vi "Sort Power Meters.vi"(0 "SG Path PM Accessor Base Array in":refnum<class "SG Path PM Accessor Base.lvclass">[](array[class]), 5 "Power Meter Base Array in":refnum<class "Power Meter Base.lvclass">[](array[class]), 11 "error in":errorcluster) -> (2 "All Present SG Path PMs Except Requested":refnum<class "SG Path PM Accessor Base.lvclass">[](array[class]), 3 "All Present PMs Except Requested":refnum<class "Power Meter Base.lvclass">[](array[class]), 4 "Requested SG Path PM Accessor":refnum<class "SG Path PM Accessor Base.lvclass">, 6 "Requested PM":refnum<class "Power Meter Base.lvclass">, 8 "Requested PM Found?":bool, 15 "error out":errorcluster)   [LabVIEW 2023, in "RFFixtureCharact.Instruments.lvlib" / "Power Meter Factory.lvclass"]
uses:
  Power Meter Factory.lvclass
  Power Meter Base/Power Meter Base.lvclass
  SG Path PM Accessor Base/SG Path PM Accessor Base.lvclass
  Power Meter Base/Power Meter Base.lvclass/Power Meter Base.ctl
  Power Meter Base/Properties/Write Active Instrument Info.vi
  Power Meter Base/Properties/Read Instrument Info Array.vi
  Common/Data Cache/Settings Dictionary/Setting Keys.vi
  Common/RFCalAndFixtureCharact.Common.lvlib
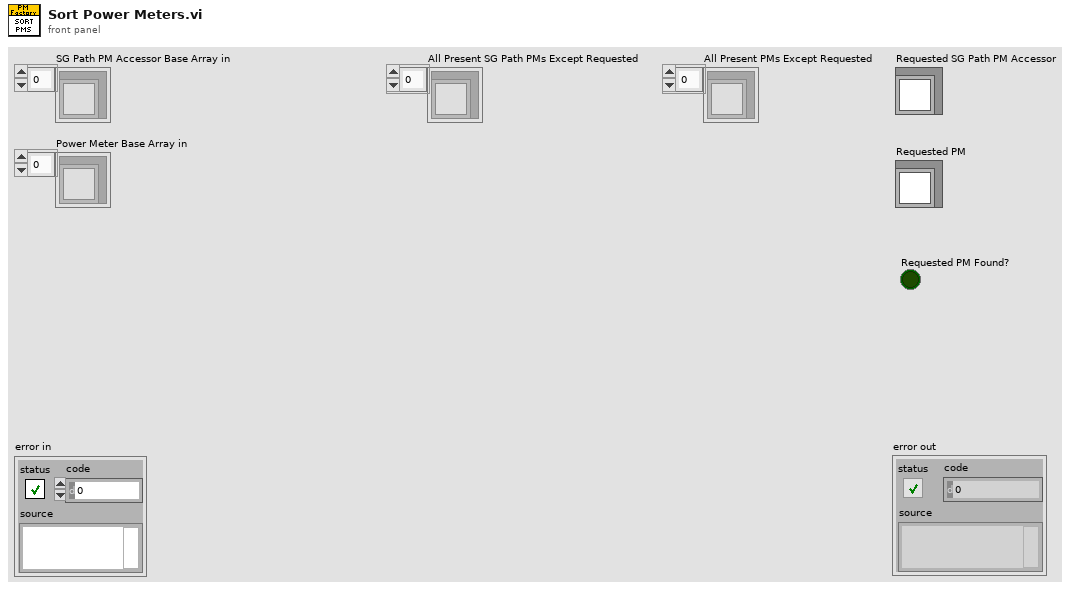
[diagram p1: front panel]
types:
  T1 = typedef "RFFixtureCharact.Instruments.lvlib/Power Meter Base.lvclass/Instrument Info.ctl" = cluster{"User Alias":string, "Resource Name":string, "Product Name":string, "Vendor Name":string}
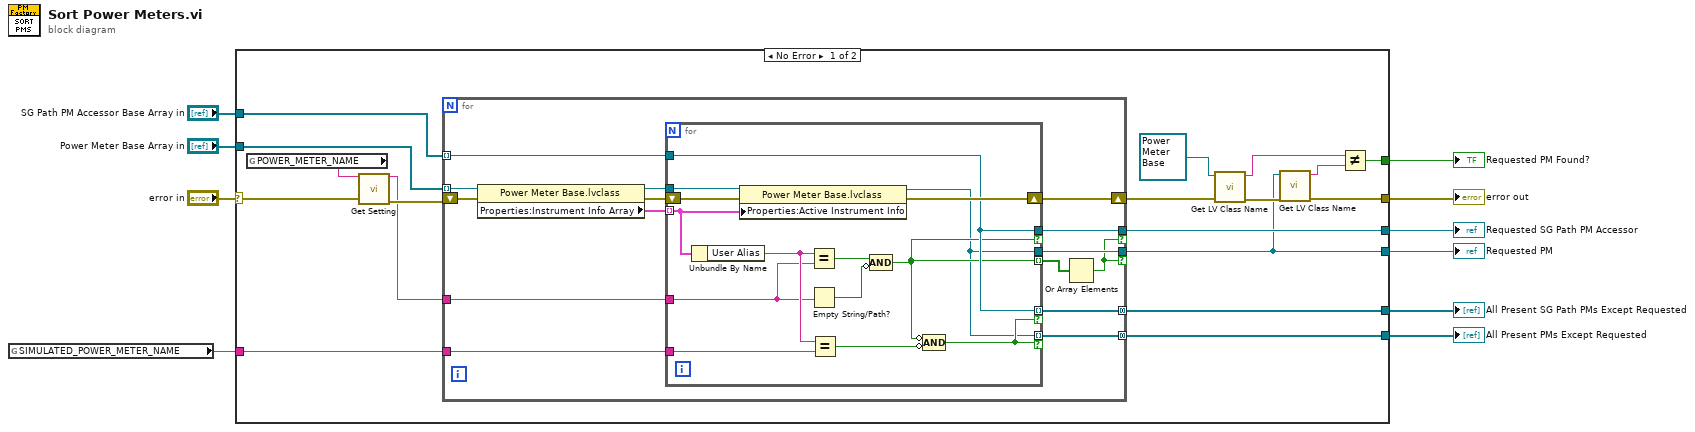
[diagram p0: block diagram]
diagram:
  n1 = global read "Setting Keys.vi" "SIMULATED_POWER_METER_NAME"() -> (w7:string)
  n2 = case shown="No Error" "error in" {
    selector: "error in" -> [w22 w58]
    tunnel: "SG Path PM Accessor Base Array in" -> [w27 _]
    tunnel: "Power Meter Base Array in" -> [w28 _]
    tunnel: [w13 w58] -> w8
    tunnel: w7 -> [w26 _]
    tunnel: [w12 _] -> w6
    tunnel: [w25 _] -> w5
    tunnel: [w24 _] -> w4
    tunnel: [w19 _] -> w3
    tunnel: [w11 _] -> w1
    frame No Error {
      n3 = global read "Setting Keys.vi" "POWER_METER_NAME"() -> (w23:string)
      n4 = call "Get Setting.vi"("Setting name"=w23, "error in (no error)"=w22) -> ("Setting value out"=w20:string, "error out"=w21:errorcluster)  [unwired: 11 in, 1 out]
      n5 = for {
        tunnel: w27 -> [w39] mode=indexing
        tunnel: w28 -> [w43] mode=indexing
        shift-right: [w31] -> w15
        shift-left: w21 -> [w42]
        tunnel: w20 -> [w38]
        tunnel: [w32] -> w12 if=w29
        tunnel: w26 -> [w36]
        tunnel: [w35] -> w25 mode=concatenating
        tunnel: [w33] -> w24 if=w29
        tunnel: [w34] -> w19 mode=concatenating
        n6 = property class="Power Meter Base.lvclass"(reference=w43, error in=w42) -> (reference out=w40:refnum<class "Power Meter Base.lvclass">, error out=w37:errorcluster, "Properties:Instrument Info Array"=w41:T1[])
        n7 = for {
          tunnel: w41 -> [w46] mode=indexing
          tunnel: w40 -> [w47]
          tunnel: w39 -> [w48]
          tunnel: w38 -> [w53]
          tunnel: [w44] -> w32 if=w45
          shift-right: [w49] -> w31
          shift-left: w37 -> [w50]
          tunnel: w36 -> [w57]
          tunnel: [w44] -> w35 mode=indexing if=w51
          tunnel: [w48] -> w33 if=w45
          tunnel: [w48] -> w34 mode=indexing if=w51
          tunnel: [w45] -> w30 mode=indexing
          n8 = Unbundle By Name(w46) -> ("User Alias"=w56:string)
          n9 = property class="Power Meter Base.lvclass"(reference=w47, error in=w50, "Properties:Active Instrument Info"=w46) -> (reference out=w44:refnum<class "Power Meter Base.lvclass">, error out=w49:errorcluster)
          n10 = Equal?(x=w56, y=w53) -> (x = y?=w55:bool)
          n11 = Empty String/Path?(string/path=w53) -> (empty?=w54:bool)
          n12 = Equal?(x=w56, y=w57) -> (x = y?=w52:bool)
          n13 = Compound Arithmetic op=AND(w55, invert w54) -> (w45:bool)
          n14 = Compound Arithmetic op=AND(invert w45, invert w52) -> (w51:bool)
        }
        n15 = Or Array Elements(Boolean array=w30) -> (logical OR=w29:bool)
      }
      n16 = call <vilib>:"Get LV Class Name.vi"("error in (no error)"=w15, "object"=refnum<class "Power Meter Base.lvclass"> refnum ("Requested PM")) -> ("error out"=w14:errorcluster, "class name"=w17:string)  [unwired: 8 in]
      n17 = call <vilib>:"Get LV Class Name.vi"("error in (no error)"=w14, "object"=w12) -> ("error out"=w13:errorcluster, "class name"=w16:string)  [unwired: 8 in]
      n18 = Not Equal?(x=w17, y=w16) -> (x != y?=w11:bool)
    }
    frame Error {
    }
  }
  "Requested PM" <- w6
  "error out" <- w8
  "All Present PMs Except Requested" <- w5
  "Requested SG Path PM Accessor" <- w4
  "All Present SG Path PMs Except Requested" <- w3
  "Requested PM Found?" <- w1
